vi "Clear Error.vi"(7 "error to clear":T1, 8 "error in (no error)":errorcluster, 11 "Interface in":refnum<class "Interface.lvclass">) -> (0 "error out":errorcluster, 1 "specific error cleared?":bool, 3 "Interface out":refnum<class "Interface.lvclass">)   [LabVIEW 2017, in "DSF Core.lvlib" / "Interface.lvclass"]
uses:
  Interface.lvclass
  Errors.ctl
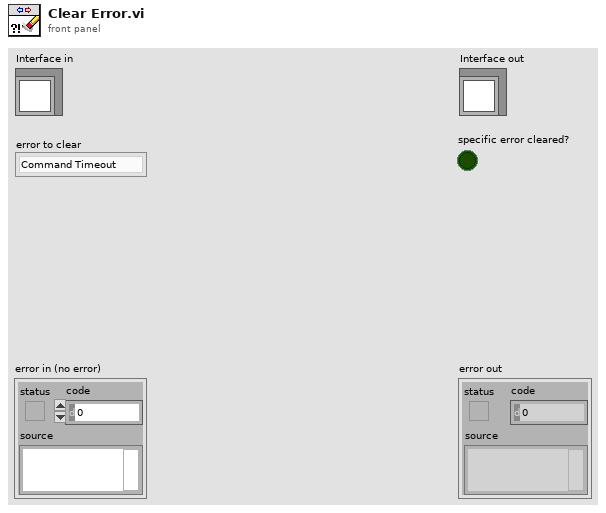
[diagram p1: front panel]
types:
  T1 = typedef "DSF Core.lvlib/Interface.lvclass/Errors.ctl" = enum16{"Command Timeout", "Response Timeout", "Error Timeout", "Invalid Response", "Invalid Response Parameters"}
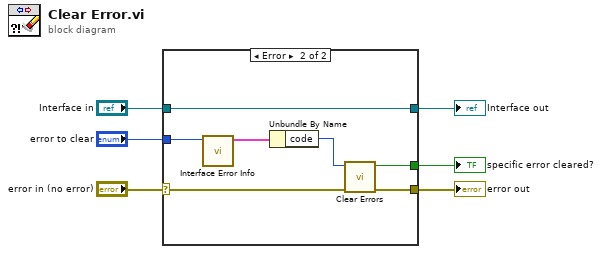
[diagram p0: block diagram]
diagram:
  n1 = case shown="Error" "error in (no error)" {
    selector: "error in (no error)" -> [w7 w12]
    tunnel: [w7 w9] -> w5
    tunnel: [w8 w15] -> w3
    tunnel: "Interface in" -> [w8 w15]
    tunnel: "error to clear" -> [_ w14]
    tunnel: [_ w10] -> w1
    frame No Error {
      # "No error to clear."
    }
    frame Error {
      n2 = call "Interface Error Info.vi"("error"=w14) -> ("error info"=w13:cluster{"code":i32, "description":string})  [unwired: 10 in]
      n3 = Unbundle By Name(w13) -> ("code"=w11:i32)
      n4 = call <vilib>:"Clear Errors.vi"("error in (no error)"=w12, "specific error code to clear (0: all)"=w11) -> ("error out"=w9:errorcluster, "specific error cleared?"=w10:bool)  [unwired: 4 in]
    }
  }
  "error out" <- w5
  "Interface out" <- w3
  "specific error cleared?" <- w1
